vi "Check_Loop_Error_FGV.vi"(5 "Case":string, 7 "VI_name":string, 8 "error in (no error)":errorcluster, 9 "queue IN":refnum<queue>, 10 "Ignore Errors":i32[](array[numeric]), 11 "Exit on Error? (F)":bool) -> (3 "Boolean":bool)   [LabVIEW 2024, in "Relay_Module.lvlib"]
doc: "ThisVI\n---------------------------------------------------\nCheck Loop Error List\n---------------------------------------------------\n-Checks the Error Code .\n-Eneque the \"Exit\" or \"Error\" message if error code in Ignore Error List."
uses:
  Relay_Module.lvlib
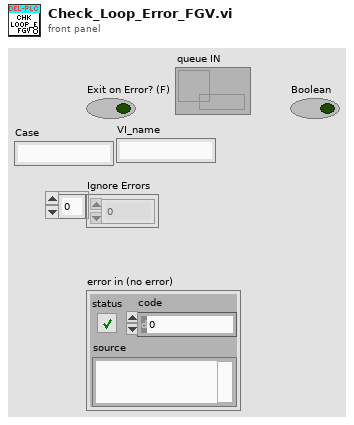
[diagram p1: front panel]
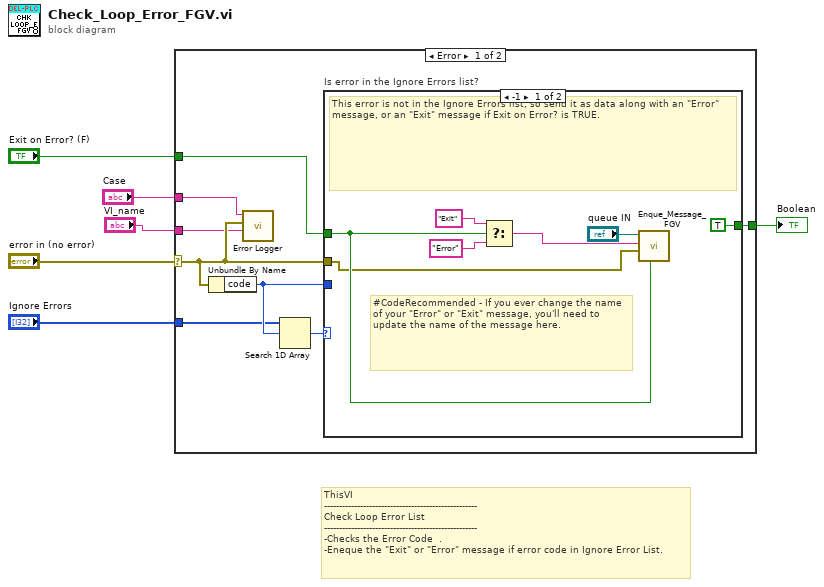
[diagram p0: block diagram]
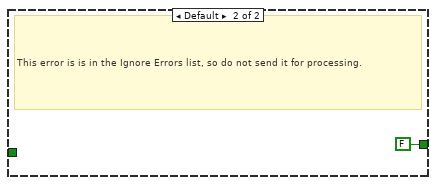
[diagram p2: hidden frame]
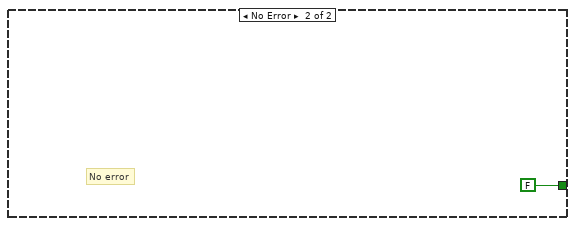
[diagram p3: hidden frame]
diagram:
  # "ThisVI\n---------------------------------------------------\nCheck Loop Error List\n---------------------------------------------------\n-Checks the Error Code  .\n-Eneque the \"Exit\" or \"Error\" message if error code in Ignore Error List."
  n1 = case shown="Error" "error in (no error)" {
    selector: "error in (no error)" -> [w9 _]
    tunnel: "Ignore Errors" -> [w12 _]
    tunnel: [w11 FALSE] -> w5
    tunnel: "Exit on Error? (F)" -> [w10 _]
    tunnel: "VI_name" -> [w8 _]
    tunnel: "Case" -> [w7 _]
    frame Error {
      n2 = Unbundle By Name(w9) -> ("code"=w13:i32)
      n3 = call "Error Logger.vi"("VI_name"=w8, "Error"=w9, "Case"=w7) -> ()  [unwired: 8 in, 1 out]
      n4 = Search 1D Array(1D array=w12, element=w13) -> (index of element=w14:i32)  [unwired: 1 in]
      n5 = case "Is error in the Ignore Errors list?" shown="-1" w14 {
        tunnel: w9 -> [w17 _]
        tunnel: w13 -> [_ _]
        tunnel: [TRUE FALSE] -> w11
        tunnel: w10 -> [w18 _]
        frame -1 {
          # "#CodeRecommended - If you ever change the name of your \"Error\" or \"Exit\" message, you'll need to update the name of the message here."
          # "This error is not in the Ignore Errors list, so send it as data along with an \"Error\" message, or an \"Exit\" message if Exit on Error? is TRUE."
          n6 = Select(t="Exit" ("Message"), s=w18, f="Error" ("Message")) -> (s? t:f=w16:string)
          n7 = call "Enque_Message_FGV.vi"("Priority"=w18, "Message Data"=w17, "Message"=w16, "queue IN"="queue IN") -> ()  [unwired: 7 in, 1 out]
        }
        frame Default {
          # "This error is is in the Ignore Errors list, so do not send it for processing."
        }
      }
    }
    frame No Error {
      # "No error"
    }
  }
  "Boolean" <- w5
